vi "MongoDB.FindandRemove.vi"(8 "error in (no error)":errorcluster, 10 "Query":string, 11 "MongoDB.Collection in":refnum<class "MongoDB.Collection.lvclass">) -> (0 "error out":errorcluster, 3 "MongoDB.Collection out":refnum<class "MongoDB.Collection.lvclass">)   [LabVIEW 2014, in "MongoDB.Collection.lvclass"]
uses:
  MongoDB.Collection.lvclass
  MongoDB.Collection.lvclass/MongoDB.Collection.ctl
  C:/Users/Richard/Documents/GitHub/mongo-labview-driver/CSharp/bin/MongoDB.Driver.Legacy.dll
  CSharp/bin/MongoDB.Driver.Legacy.dll
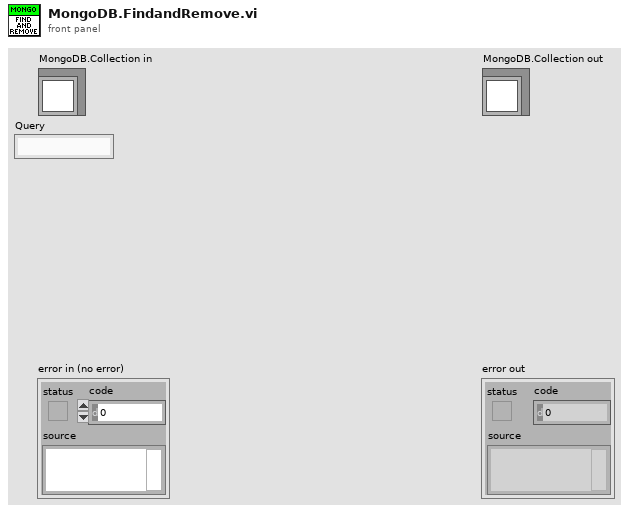
[diagram p1: front panel]
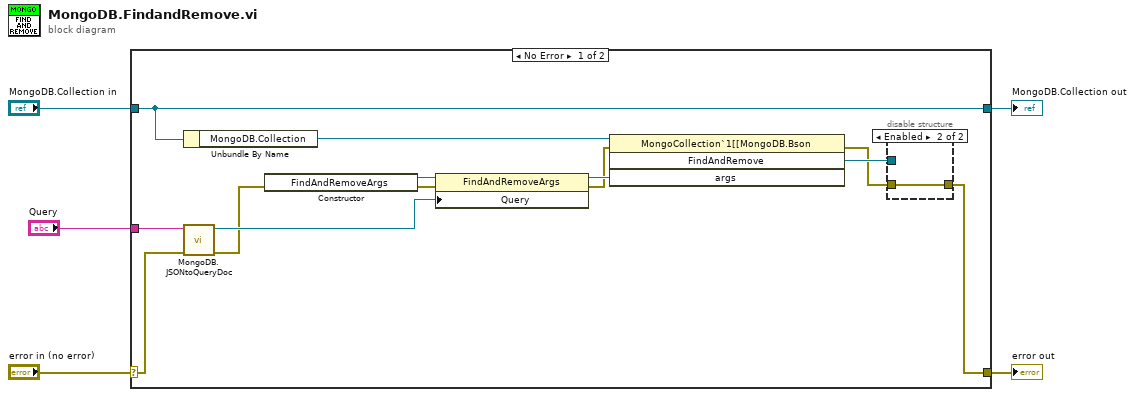
[diagram p0: block diagram]
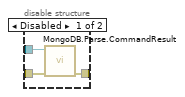
[diagram p2: hidden frame]
diagram:
  n1 = case shown="No Error" "error in (no error)" {
    selector: "error in (no error)" -> [w7 w24]
    tunnel: [w14 w24] -> w4
    tunnel: [w18 w23] -> w2
    tunnel: "MongoDB.Collection in" -> [w18 w23]
    tunnel: "Query" -> [w11 _]
    frame No Error {
      n2 = Unbundle By Name(w18) -> ("MongoDB.Collection"=w17:refnum<k24>)
      n3 = call "MongoDB.JSONtoQueryDoc.vi"("error in (no error)"=w7, "JSON Query String"=w11) -> ("error out"=w6:errorcluster, ".NET Refnum out"=w13:refnum<k24>)  [unwired: 8 in]
      n4 = constructor class="FindAndRemoveArgs"(error in=w6) -> (reference out=w12:refnum<k24>, error out=w9:errorcluster)  [unwired: 2 in, 1 out]
      n5 = property class="FindAndRemoveArgs"(reference=w12, error in=w9, "Query"=w13) -> (reference out=w10:refnum<k24>, error out=w8:errorcluster)
      n6 = invoke class="MongoCollection`1[[MongoDB.Bson" method="FindAndRemove"(reference=w17, error in=w8, "args"=w10) -> (error out=w15:errorcluster, "FindAndRemove"=w16:refnum<k24>)  [unwired: 1 in, 2 out]
      n7 = disable-structure shown="Enabled" {
        disable-tunnel: w16 -> [w21 _]
        disable-tunnel: w15 -> [w20 w22]
        disable-tunnel: [w19 w22] -> w14
        frame Disabled {
          n8 = call "MongoDB.Parse.CommandResult.vi"("error in (no error)"=w20, "MongoDB.Command.Result"=w21) -> ("error out"=w19:errorcluster)  [unwired: 9 in]
        }
        frame Enabled {
        }
      }
    }
    frame Error {
    }
  }
  "error out" <- w4
  "MongoDB.Collection out" <- w2
